vi "ProducerConsumerEvents 2.vi"() -> ()   [LabVIEW 2010]
doc: "Use this template to build a producer/consumer design pattern with events to produce queue items. Use this design pattern instead of the User Interface Event Handler pattern for user interfaces when you want to execute code asynchronously in response to an event without slowing the user interface responsiveness."
panel:
  in  "Queue Event":bool
  in  "stop":bool
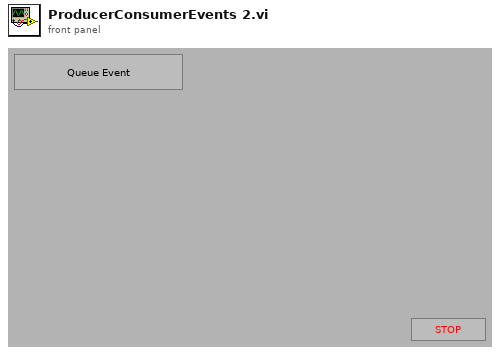
[diagram p1: front panel]
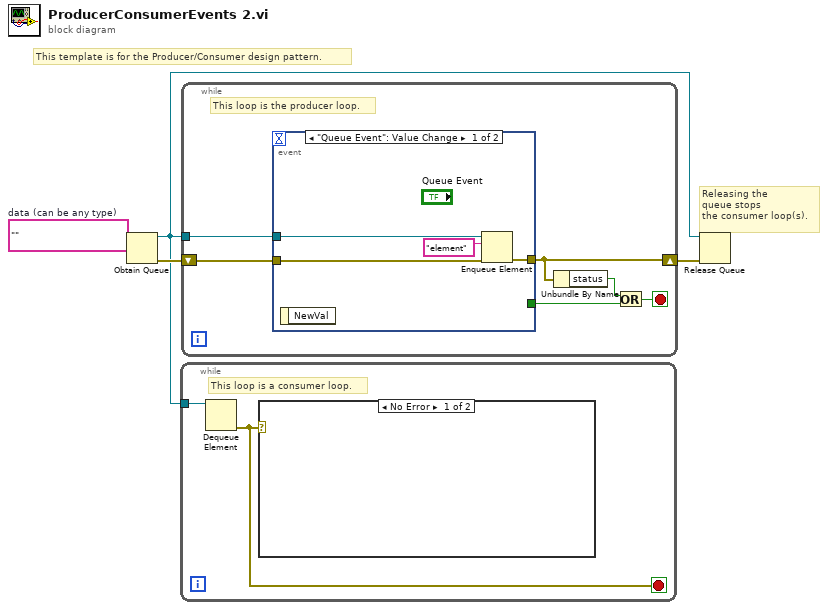
[diagram p0: block diagram]
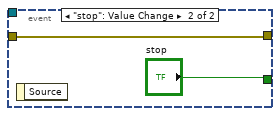
[diagram p3: hidden frame]
diagram:
  w2 = ""  # data (can be any type)
  # "Releasing the\nqueue stops\nthe consumer loop(s)."
  # "This template is for the Producer/Consumer design pattern."
  n1 = Obtain Queue(element data type=w2) -> (queue out=w1:refnum<queue>, error out=w4:errorcluster)  [unwired: 4 in, 1 out]
  n2 = while {
    tunnel: w1 -> [w6]
    stop <- w5 stop-if-true
    # "This loop is a consumer loop."
    n3 = Dequeue Element(queue=w6) -> (error out=w5:errorcluster)  [unwired: 2 in, 3 out]
    n4 = case shown="No Error" w5 {
      frame No Error {
      }
      frame Error {
      }
    }
  }
  n5 = while {
    shift-right: [w8] -> w3
    shift-left: w4 -> [w11]
    tunnel: w1 -> [w12]
    stop <- w9 stop-if-true
    # "This loop is the producer loop."
    n6 = event shown="[0] \"Queue Event\": Value Change" {
      selector: _ -> [_ _]
      dyn-events: _ -> [_ _]
      timeout: _ -> [_ _]
      tunnel: w12 -> [w16 _]
      tunnel: w11 -> [w15 w17]
      tunnel: [w14 w17] -> w8
      tunnel: [_ "stop"] -> w10
      event "Queue Event": Value Change {
        n7 = event-data() -> ()  [unwired: 1 in, 1 out]
        n8 = Enqueue Element(queue=w16, element="element", error in (no error)=w15) -> (error out=w14:errorcluster)  [unwired: 1 in, 2 out]
      }
      event "stop": Value Change {
        n9 = event-data() -> ()  [unwired: 1 in, 1 out]
      }
    }
    n10 = Unbundle By Name(w8) -> ("status"=w7:bool)
    n11 = Or(x=w7, y=w10) -> (x .or. y?=w9:bool)
  }
  n12 = Release Queue(queue=w1, error in (no error)=w3) -> ()  [unwired: 1 in, 3 out]
